vi "DrawSprites.vi"(8 "error in (no error)":errorcluster, 10 "Sprites in":refnum<class "RT_Sprite.lvclass">[](array[class]), 11 "Engine in":refnum<class "Engine.lvclass">) -> (0 "error out":errorcluster, 3 "Engine out":refnum<class "Engine.lvclass">)   [LabVIEW 2019, in "RT_Game.lvlib" / "Engine.lvclass"]
uses:
  Engine.lvclass
  RT_Sprite/RT_Sprite.lvclass
  C:/Users/FreshBob/Dropbox/VIs/myRIO_GameConsole/RT/RT_Game/GameObject/GameObject.lvclass
  Engine.lvclass/Engine.ctl
  FPGA/Sprite/SpriteData.ctl
  GameObject/GameObject.lvclass/GameObject.ctl
  RT_Sprite/RT_Sprite.lvclass/RT_Sprite.ctl
  GameObject/Read position.vi
  GameObject/Read size.vi
  GameObject/Read IsActive.vi
  RT_Sprite/Read TransparentColor.vi
  <vilib>/Utility/error.llb/Error Cluster From Error Code.vi
  <vilib>/rvi/errors/niLvFpgaAdjustHostInterfaceError.vi
  <vilib>/rvi/interface/nirviReadWriteControl/nirviReadWriteControl.xnode
  FPGA_Interface.ctl
  FPGA Bitfiles/myriogameconsole_FPGATarget_Main_ntsPRcBZGxk.lvbitx
  FPGA/Sprite/Sprite.lvlib
  NiFpgaLv.dll
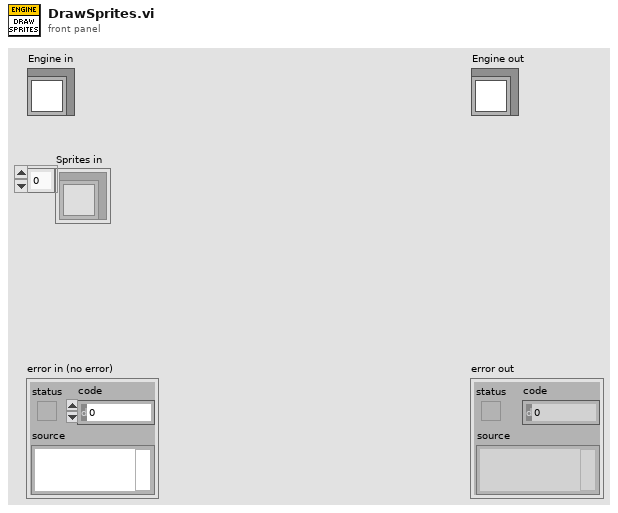
[diagram p1: front panel]
types:
  T1 = typedef "Sprite.lvlib/SpriteData.ctl" = cluster{"Pos_X":i16, "Pos_Y":i16, "Width":i16, "Height":i16, "BufferIndex":i16, "TransparencyColor":fxp<+,3,3>}
  T2 = typedef "FPGA_Interface.ctl" = refnum<k20>
  T3 = typedef "RT_Game.lvlib/Game.lvclass/Coordinate.ctl" = cluster{"x":dbl, "y":dbl}
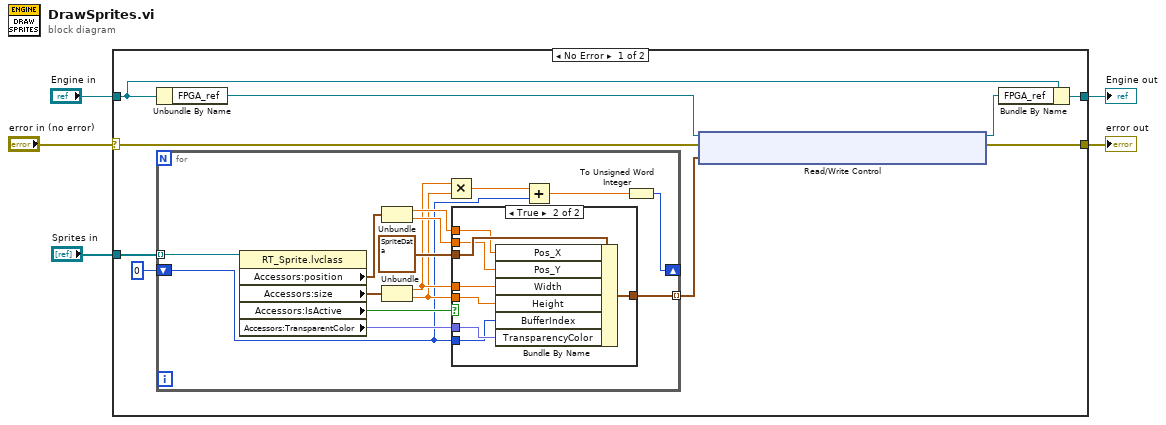
[diagram p0: block diagram]
diagram:
  n1 = case shown="No Error" "error in (no error)" {
    selector: "error in (no error)" -> [w7 w40]
    tunnel: [w6 w40] -> w4
    tunnel: [w9 w39] -> w2
    tunnel: "Engine in" -> [w11 w39]
    tunnel: "Sprites in" -> [w12 _]
    frame No Error {
      n2 = Unbundle By Name(w11) -> ("FPGA_ref"=w10:T2)
      n3 = for {
        tunnel: [w27] -> w13 mode=indexing
        tunnel: w12 -> [w28] mode=indexing
        shift-right: [w15] -> _
        shift-left: u16 0 ("BufferIndex") -> [w16]
        n4 = property class="RT_Sprite.lvclass"(reference=w28) -> ("Accessors:position"=w26:T3, "Accessors:size"=w24:T3, "Accessors:IsActive"=w18:bool, "Accessors:TransparentColor"=w17:fxp<+,3,3>)  [unwired: 1 in, 2 out]
        n5 = Unbundle(w26) -> ("x"=w23:dbl, "y"=w25:dbl)
        n6 = Unbundle(w24) -> ("x"=w22:dbl, "y"=w21:dbl)
        n7 = Multiply(x=w22, y=w21) -> (x*y=w19:dbl)
        n8 = case shown="True" w18 {
          tunnel: T1 {"Pos_X"=0, "Pos_Y"=0, "Width"=0, "Height"=0, "BufferIndex"=0, "TransparencyColor"=0.0} ("Sprite1") -> [w30 w38]
          tunnel: [w30 w37] -> w27
          tunnel: w25 -> [_ w36]
          tunnel: w23 -> [_ w35]
          tunnel: w22 -> [_ w34]
          tunnel: w21 -> [_ w33]
          tunnel: w17 -> [_ w32]
          tunnel: w16 -> [_ w31]
          frame False {
          }
          frame True {
            n9 = Bundle By Name(cluster=w38, "Pos_X"=w35, "Pos_Y"=w36, "Width"=w34, "Height"=w33, "BufferIndex"=w31, "TransparencyColor"=w32) -> (w37:T1)
          }
        }
        n10 = Add(x=w19, y=w16) -> (x+y=w20:dbl)
        n11 = To Unsigned Word Integer(number=w20) -> (unsigned 16bit integer=w15:u16)
      }
      n12 = xnode "Read/Write Control"("FPGA VI Reference In"=w10, "error in"=w7, "Sprites"=w13) -> ("FPGA VI Reference Out"=w8:T2, "error out"=w6:errorcluster)
      n13 = Bundle By Name(cluster=w11, "FPGA_ref"=w8) -> (w9:refnum<class "Engine.lvclass">)
    }
    frame Error {
    }
  }
  "error out" <- w4
  "Engine out" <- w2
